vi "setBlockStatistics.vi"(1 "PostProDataPerBlock in":T1[][](array[typedef])) -> (0 "PostProDataPerBlock out":T1[][](array[typedef]))   [LabVIEW 2017]
uses:
  Controls/postProData.ctl
  Controls/U.ctl
  Globals/measurementGlobal.vi
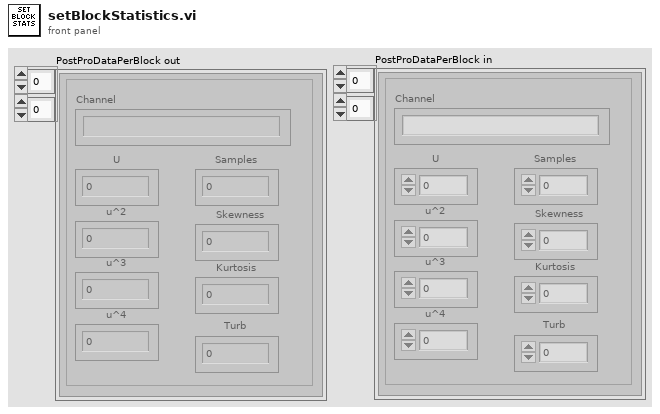
[diagram p1: front panel]
types:
  T1 = typedef "postProData.ctl" = cluster{"Channel":string, "Samples":i32, "U":dbl, "u^2":dbl, "u^3":dbl, "u^4":dbl, "Kurtosis":dbl, "Skewness":dbl, "Turb":dbl}
  T2 = typedef "chanData.ctl" = cluster{"Raw Data":dbl[], "Channel Name":string}
  T3 = typedef "U.ctl" = cluster{"Samples":dbl, "U":dbl, "U2":dbl, "U3":dbl, "U4":dbl}
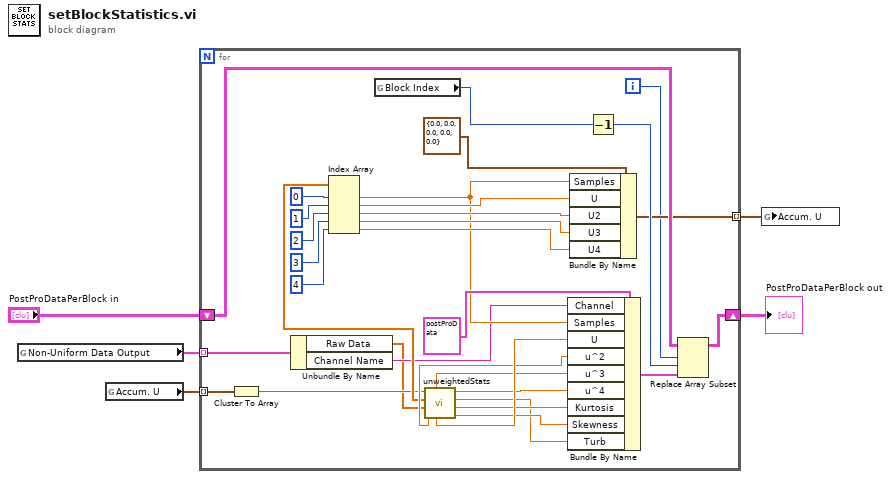
[diagram p0: block diagram]
diagram:
  n1 = global read "measurementGlobal.vi" "Non-Uniform Data Output"() -> (w2:T2[])
  n2 = global read "measurementGlobal.vi" "Accum. U"() -> (w1:T3[])
  n3 = for {
    shift-right: [w37] -> w5
    shift-left: "PostProDataPerBlock in" -> [w36]
    tunnel: [w13] -> w3 mode=indexing
    tunnel: w1 -> [w8] mode=indexing
    tunnel: w2 -> [w10] mode=indexing
    i -> [w11]
    n4 = Cluster To Array(cluster=w8) -> (array=w7:dbl[])
    n5 = Unbundle By Name(w10) -> ("Raw Data"=w6:dbl[], "Channel Name"=w9:string)
    n6 = global read "measurementGlobal.vi" "Block Index"() -> (w33:i32)
    n7 = call "unweightedStats.vi"("U"=w6, "Data Shift Input"=w7) -> ("Skew"=w29:dbl, "Kurt"=w28:dbl, "u'/U"=w27:dbl, "u^4"=w26:dbl, "U"=w31:dbl, "u^3"=w25:dbl, "u^2"=w30:dbl, "Data Shift Output"=w23:dbl[])
    n8 = Index Array(array=w23, index #1=0 ("index"), index #2=1 ("index"), index #3=2 ("index"), index #4=3 ("index"), index #5=4 ("index")) -> (element #1=w12:dbl, element #2=w17:dbl, element #3=w16:dbl, element #4=w15:dbl, element #5=w14:dbl)
    n9 = Bundle By Name(cluster=T1 {"Channel"="", "Samples"=0, "U"=0.0, "u^2"=0.0, "u^3"=0.0, "u^4"=0.0, "Kurtosis"=0.0, "Skewness"=0.0, "Turb"=0.0} ("Post Pro Data"), "Channel"=w9, "Samples"=w12, "U"=w31, "u^2"=w30, "u^3"=w25, "u^4"=w26, "Kurtosis"=w28, "Skewness"=w29, "Turb"=w27) -> (w34:T1)
    n10 = Bundle By Name(cluster=T3 {"Samples"=0.0, "U"=0.0, "U2"=0.0, "U3"=0.0, "U4"=0.0} ("Accum. U"), "Samples"=w12, "U"=w17, "U2"=w16, "U3"=w15, "U4"=w14) -> (w13:T3)
    n11 = Decrement(x=w33) -> (x-1=w32:i32)
    n12 = Replace Array Subset(array=w36, new element=w34, index (row)=w11, index (col)=w32) -> (w37:T1[][])
  }
  "PostProDataPerBlock out" <- w5
  n13 = global write "measurementGlobal.vi" "Accum. U"(w3) -> ()
